vi "Obtain Request Events.vi"(8 "error in (no error)":errorcluster, 10 "Create New?":bool) -> (0 "error out":errorcluster, 2 "FlexiFlowInterface Request Events":T1)   [LabVIEW 2024, in "FlexiFlowInterface.lvlib"]
doc: "This VI Obtains/Creates the Requests events that will be used for other modules to communicate with the module that owns this VI. These Requests events will be accessed only via Public API methods for this module.\n\n<b>NOTE</b>: The contents of this VI are automatically generated and modified by the <b>Tools > Delacor > DQMH</b> utilities. Consider using those utilities instead of making your own modifications to this VI.\n_____\nBased on Delacor QMH Project Template 3.1.0.34."
uses:
  FlexiFlowInterface.lvlib
  Request Events--cluster.ctl
  Stop Argument--cluster.ctl
  Show Panel Argument--cluster.ctl
  Hide Panel Argument--cluster.ctl
  Get Module Execution Status Argument--cluster.ctl
  Show Diagram Argument--cluster.ctl
  Change Panel Argument--cluster.ctl
  <vilib>/MGI/Panel Manager/Panel/Panel/Panel.lvclass
  Start Modbus Polling Helper Loop Argument--cluster.ctl
  Sleep Modbus Polling Helper Loop Argument--cluster.ctl
  Wake Connection Helper Loop Argument--cluster.ctl
  Sleep Connection Helper Loop Argument--cluster.ctl
  Initialise Modbus Connections Argument--cluster.ctl
  Read Fmeasure Argument--cluster.ctl
  FlexiFlowDevice--enum.ctl
  Set Modbus Configuration Argument--cluster.ctl
  Modbus TCP Connection Settings--cluster.ctl
  Wink Devices Argument--cluster.ctl
  Read All FlexiFlow Device States Argument--cluster.ctl
  Wink Device Argument--cluster.ctl
  Set Control Function Argument--cluster.ctl
  Modbus Flexi-Flow API/Control Function Values--enum.ctl
  Set Flow Setpoint Argument--cluster.ctl
  Set Backpressure Setpoint Argument--cluster.ctl
  Set Forward Pressure SP Argument--cluster.ctl
  Set Capacity Unit Argument--cluster.ctl
  Capacity unit--text ring.ctl
  Set Flow Capacity Unit Argument--cluster.ctl
  Modbus Flexi-Flow API/Capacity Units (Standard Volume Flow).ctl
  Set Setpoint Slope Argument--cluster.ctl
  Set Counter Settings Argument--cluster.ctl
  Counter Settings--cluster.ctl
  Modbus Flexi-Flow API/Counter Setpoint Mode--enum.ctl
  Modbus Flexi-Flow API/Counter Modes--enum.ctl
  Reset All Device Counters Argument--cluster.ctl
  Read Device User Tag Argument--cluster.ctl
  Set Device User Tag Argument--cluster.ctl
  Read Counter Unit Argument--cluster.ctl
  Set Control Mode Argument--cluster.ctl
  Modbus Flexi-Flow API/Control Mode--enum.ctl
  Get Device Configuration Argument--cluster.ctl
  Modbus Flexi-Flow API/Bronkhorst Flexi-Flow ModbusTCP API.lvlib
  Anode/Anode.lvlib
panel:
  # "NOTE: The contents of this VI are automatically generated and modified by the Tools > Delacor > DQMH utilities. Consider using those utilities instead of making your own modifications to this VI."
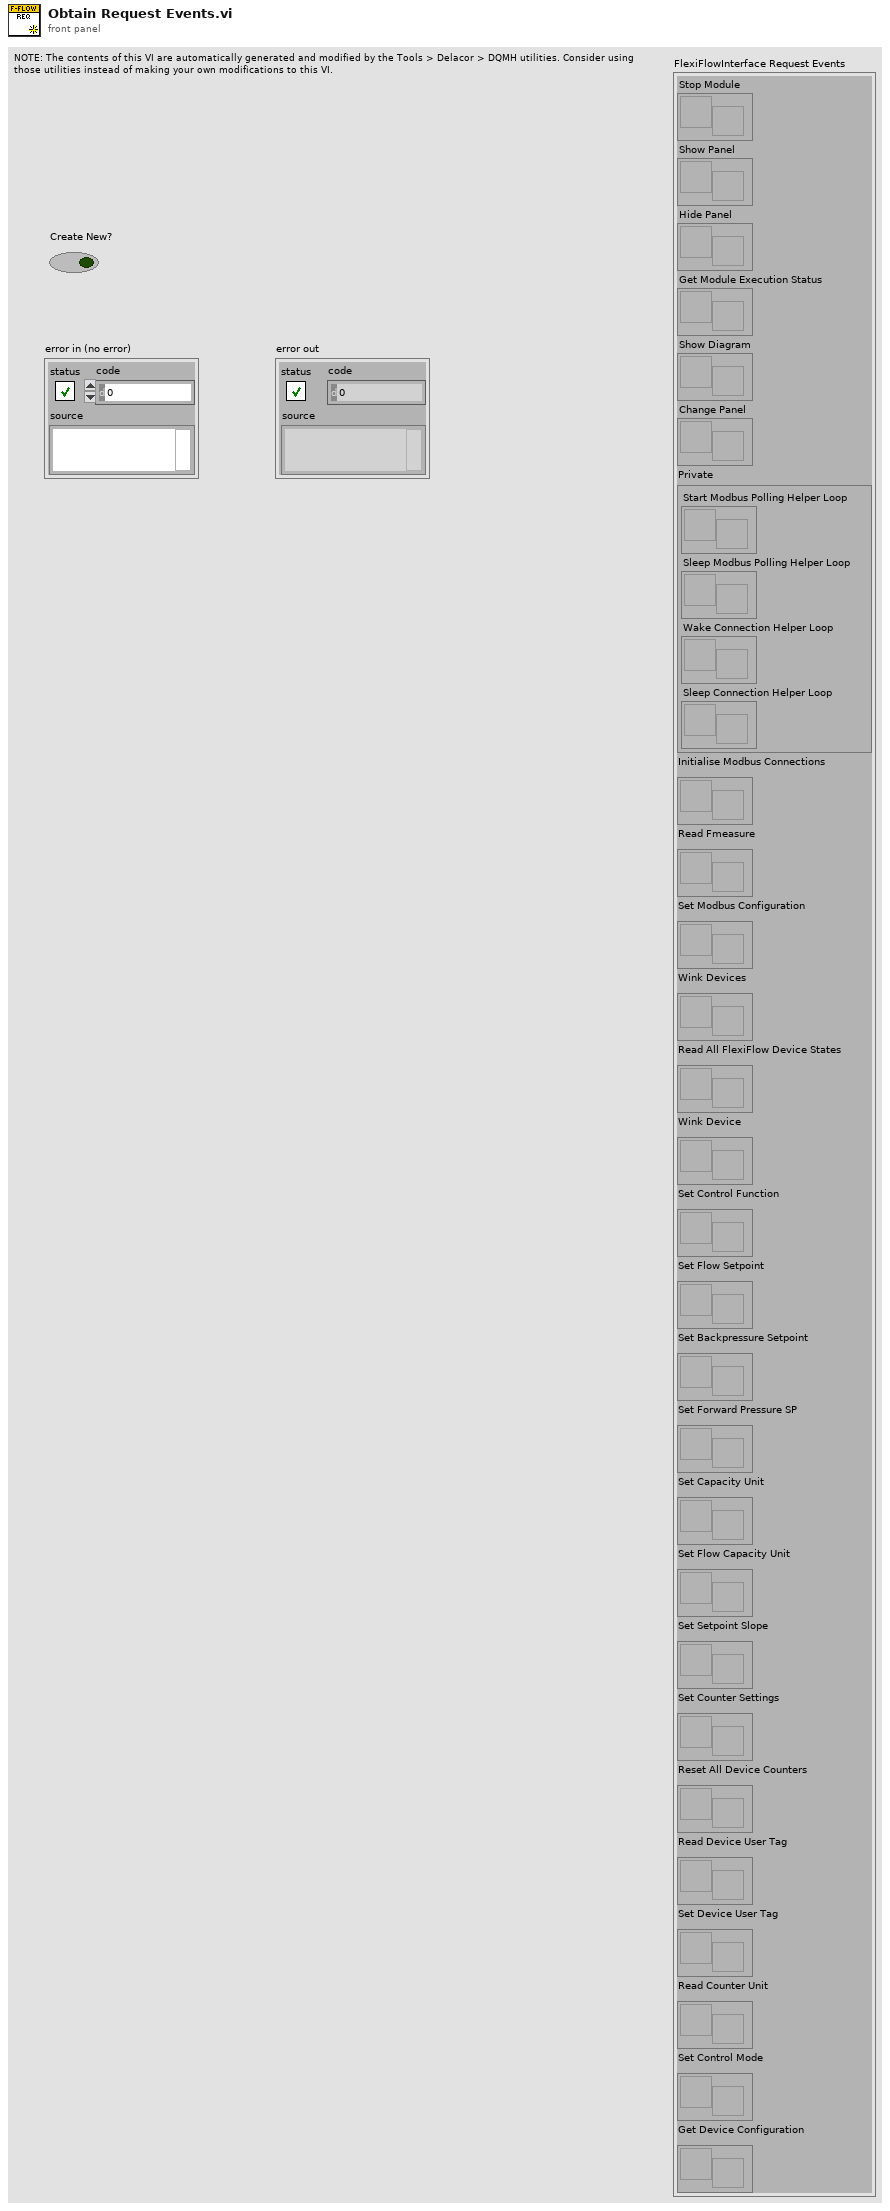
[diagram p1: front panel]
types:
  T1 = typedef "FlexiFlowInterface.lvlib/Request Events--cluster.ctl" = cluster{"Stop Module":refnum<user-event>, "Show Panel":refnum<user-event>, "Hide Panel":refnum<user-event>, "Get Module Execution Status":refnum<user-event>, "Show Diagram":refnum<user-event>, "Change Panel":refnum<user-event>, "Private":cluster{"Start Modbus Polling Helper Loop":refnum<user-event>, "Sleep Modbus Polling Helper Loop":refnum<user-event>, "Wake Connection Helper Loop":refnum<user-event>, "Sleep Connection Helper Loop":refnum<user-event>}, "Initialise Modbus Connections":refnum<user-event>, "Read Fmeasure":refnum<user-event>, "Set Modbus Configuration":refnum<user-event>, "Wink Devices":refnum<user-event>, "Read All FlexiFlow Device States":refnum<user-event>, "Wink Device":refnum<user-event>, "Set Control Function":refnum<user-event>, "Set Flow Setpoint":refnum<user-event>, "Set Backpressure Setpoint":refnum<user-event>, "Set Forward Pressure SP":refnum<user-event>, "Set Capacity Unit":refnum<user-event>, "Set Flow Capacity Unit":refnum<user-event>, "Set Setpoint Slope":refnum<user-event>, "Set Counter Settings":refnum<user-event>, "Reset All Device Counters":refnum<user-event>, "Read Device User Tag":refnum<user-event>, "Set Device User Tag":refnum<user-event>, "Read Counter Unit":refnum<user-event>, "Set Control Mode":refnum<user-event>, "Get Device Configuration":refnum<user-event>}
  T2 = typedef "FlexiFlowInterface.lvlib/Sleep Connection Helper Loop Argument--cluster.ctl" = cluster{"Boolean":bool}
  T3 = typedef "FlexiFlowInterface.lvlib/Wake Connection Helper Loop Argument--cluster.ctl" = cluster{"Boolean":bool}
  T4 = typedef "FlexiFlowInterface.lvlib/Get Device Configuration Argument--cluster.ctl" = cluster{"Device":T5}
  T5 = typedef "FlexiFlowInterface.lvlib/FlexiFlowDevice--enum.ctl" = enum16{"Hydrogen Inlet", "Nitrogen Inlet", "Cathode Outlet", "Anode Outlet"}
  T6 = typedef "FlexiFlowInterface.lvlib/Set Control Mode Argument--cluster.ctl" = cluster{"Device":T5, "Control Mode":T7}
  T7 = typedef "Bronkhorst Flexi-Flow ModbusTCP API.lvlib/Control Mode--enum.ctl" = u16
  T8 = typedef "FlexiFlowInterface.lvlib/Read Counter Unit Argument--cluster.ctl" = cluster{"Device":T5}
  T9 = typedef "FlexiFlowInterface.lvlib/Set Device User Tag Argument--cluster.ctl" = cluster{"Device":T5, "User Tag":string}
  T10 = typedef "FlexiFlowInterface.lvlib/Read Device User Tag Argument--cluster.ctl" = cluster{"Device":T5}
  T11 = typedef "FlexiFlowInterface.lvlib/Reset All Device Counters Argument--cluster.ctl" = cluster{"Boolean":bool}
  T12 = typedef "FlexiFlowInterface.lvlib/Set Counter Settings Argument--cluster.ctl" = cluster{"Device":T5, "Counter Settings":T13}
  T13 = typedef "FlexiFlowInterface.lvlib/Counter Settings--cluster.ctl" = cluster{"Counter Setpoint Mode":T14, "Counter Limit":sgl, "Unit":string, "Counter Mode":T15, "Counter New Setpoint":u16}
  T14 = typedef "Bronkhorst Flexi-Flow ModbusTCP API.lvlib/Counter Setpoint Mode--enum.ctl" = enum16{"No setpoint change (default)", "Change setpoint to Counter new setpoint"}
  T15 = typedef "Bronkhorst Flexi-Flow ModbusTCP API.lvlib/Counter Modes--enum.ctl" = enum16{"Counter off (default)", "Counting up continuously", "Counting up until limit reached"}
  T16 = typedef "FlexiFlowInterface.lvlib/Set Setpoint Slope Argument--cluster.ctl" = cluster{"Setpoint Slope":u16, "Device":T5}
  T17 = typedef "FlexiFlowInterface.lvlib/Set Flow Capacity Unit Argument--cluster.ctl" = cluster{"Device":T5, "Standard Volume Flow":T18}
  T18 = typedef "Bronkhorst Flexi-Flow ModbusTCP API.lvlib/Capacity Units (Standard Volume Flow).ctl" = u16
  T19 = typedef "FlexiFlowInterface.lvlib/Set Capacity Unit Argument--cluster.ctl" = cluster{"Device":T5, "Mass Flow":T20}
  T20 = typedef "Anode.lvlib/Capacity unit--text ring.ctl" = u16
  T21 = typedef "FlexiFlowInterface.lvlib/Set Forward Pressure SP Argument--cluster.ctl" = cluster{"Device":T5, "Pressure SP":dbl}
  T22 = typedef "FlexiFlowInterface.lvlib/Set Backpressure Setpoint Argument--cluster.ctl" = cluster{"Device":T5, "Backpressure SP":dbl}
  T23 = typedef "FlexiFlowInterface.lvlib/Set Flow Setpoint Argument--cluster.ctl" = cluster{"Device":T5, "Setpoint Value":dbl}
  T24 = typedef "FlexiFlowInterface.lvlib/Set Control Function Argument--cluster.ctl" = cluster{"Device":T5, "Function":T25}
  T25 = typedef "Bronkhorst Flexi-Flow ModbusTCP API.lvlib/Control Function Values--enum.ctl" = enum16{"Flow", "Upstream pressure", "Downstream pressure", "Flow with upstream pressure limit", "Flow with downstream pressure limit", "Upstream pressure with flow limit", "Downstream pressure with flow limit"}
  T26 = typedef "FlexiFlowInterface.lvlib/Wink Device Argument--cluster.ctl" = cluster{"Device":T5}
  T27 = typedef "FlexiFlowInterface.lvlib/Read All FlexiFlow Device States Argument--cluster.ctl" = cluster{"Boolean":bool}
  T28 = typedef "FlexiFlowInterface.lvlib/Wink Devices Argument--cluster.ctl" = cluster{"Boolean":bool}
  T29 = typedef "FlexiFlowInterface.lvlib/Set Modbus Configuration Argument--cluster.ctl" = cluster{"Device":T5, "Modbus TCP Connection":T30}
  T30 = typedef "FlexiFlowInterface.lvlib/Modbus TCP Connection Settings--cluster.ctl" = cluster{"Label":string, "Slave ID (255)":u8, "IP Address":string, "Port (502)":u16, "Timeout (10000)":i32}
  T31 = typedef "FlexiFlowInterface.lvlib/Read Fmeasure Argument--cluster.ctl" = cluster{"Device":T5}
  T32 = typedef "FlexiFlowInterface.lvlib/Initialise Modbus Connections Argument--cluster.ctl" = cluster{"Boolean":bool}
  T33 = typedef "FlexiFlowInterface.lvlib/Sleep Modbus Polling Helper Loop Argument--cluster.ctl" = cluster{"Boolean":bool}
  T34 = typedef "FlexiFlowInterface.lvlib/Start Modbus Polling Helper Loop Argument--cluster.ctl" = cluster{"Boolean":bool}
  T35 = typedef "FlexiFlowInterface.lvlib/Change Panel Argument--cluster.ctl" = cluster{"New Panel":refnum<class "Panel.lvclass">}
  T36 = typedef "FlexiFlowInterface.lvlib/Hide Panel Argument--cluster.ctl" = cluster{"Hide Panel?":bool}
  T37 = typedef "FlexiFlowInterface.lvlib/Show Panel Argument--cluster.ctl" = cluster{"Show Panel?":bool}
  T38 = typedef "FlexiFlowInterface.lvlib/Show Diagram Argument--cluster.ctl" = cluster{"Debug?":bool}
  T39 = typedef "FlexiFlowInterface.lvlib/Get Module Execution Status Argument--cluster.ctl" = cluster{"Running?":bool}
  T40 = typedef "FlexiFlowInterface.lvlib/Stop Argument--cluster.ctl" = cluster{"Origin":string, "Exit via Stop Module Req?":bool, "Wait for Module to stop?":bool}
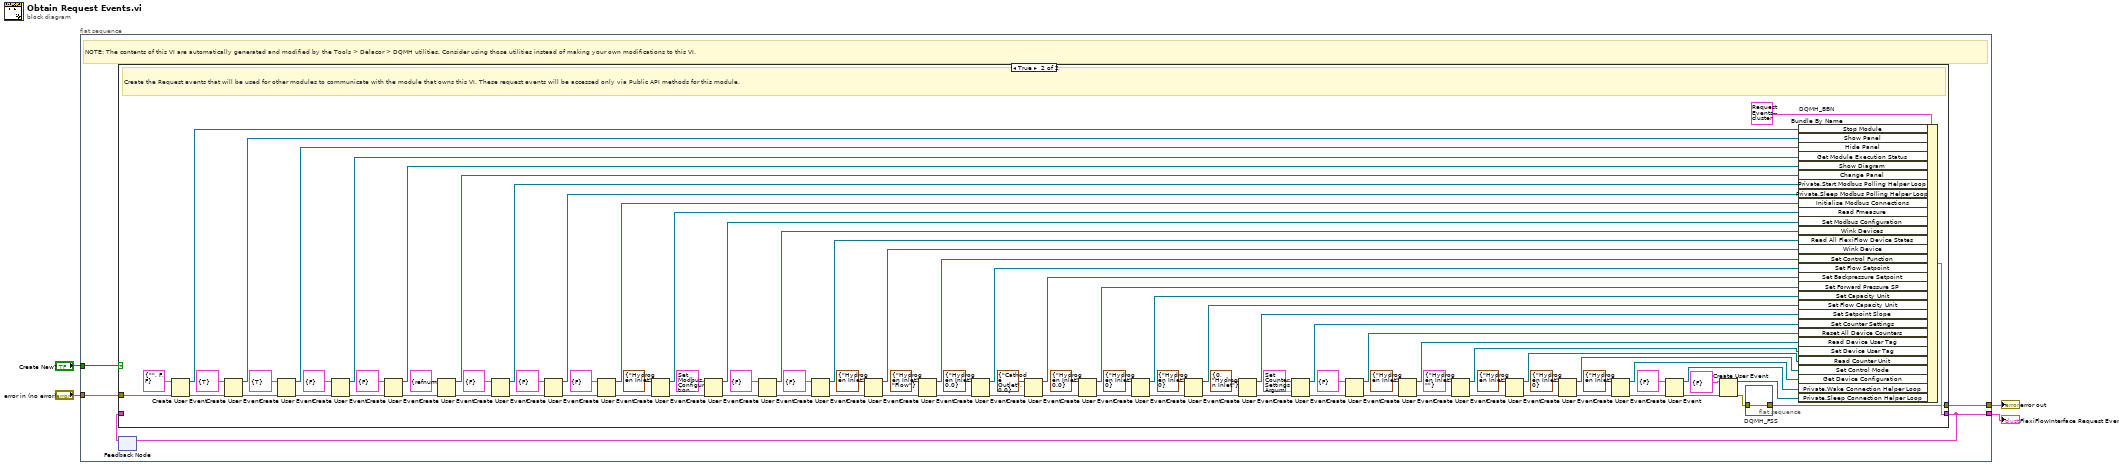
[diagram p0: block diagram]
diagram:
  n1 = flat-sequence {
    tunnel: [w9] -> w4
    tunnel: "error in (no error)" -> [w8]
    tunnel: [w6] -> w2
    tunnel: "Create New?" -> [w5]
    frame #0 {
      # "NOTE: The contents of this VI are automatically generated and modified by the Tools > Delacor > DQMH utilities. Consider using those utilities instead of making your own modifications to this VI."
      n2 = feedback #1() -> (w7:T1)  [unwired: 1 in]
      n3 = case shown="True" w5 {
        tunnel: [w10 w95] -> w9
        tunnel: w8 -> [w10 w105]
        tunnel: [w11 w102] -> w6
        tunnel: w7 -> [w11 _]
        frame False {
          # "Obtain the Request events that were created in a previous call to this VI."
        }
        frame True {
          # "Create the Request events that will be used for other modules to communicate with the module that owns this VI. These request events will be accessed only via Public API methods for this module."
          n4 = Create User Event(user event datatype=T40 {"Origin"="", "Exit via Stop Module Req?"=FALSE, "Wait for Module to stop?"=FALSE} ("Stop Argument"), error in=w105) -> (user event=w103:refnum<user-event>, error out=w100:errorcluster)
          n5 = Create User Event(user event datatype=T37 {"Show Panel?"=TRUE} ("Show Panel Argument"), error in=w100) -> (user event=w99:refnum<user-event>, error out=w98:errorcluster)
          n6 = Create User Event(user event datatype=T36 {"Hide Panel?"=TRUE} ("Hide Panel Argument"), error in=w98) -> (user event=w97:refnum<user-event>, error out=w96:errorcluster)
          n7 = Create User Event(user event datatype=T39 {"Running?"=FALSE} ("Get Module Execution Status Argument"), error in=w96) -> (user event=w93:refnum<user-event>, error out=w94:errorcluster)
          n8 = Create User Event(user event datatype=T38 {"Debug?"=FALSE} ("Show Diagram Argument"), error in=w94) -> (user event=w90:refnum<user-event>, error out=w91:errorcluster)
          n9 = Create User Event(user event datatype=T35 {"New Panel"=refnum} ("Change Panel Argument"), error in=w91) -> (user event=w85:refnum<user-event>, error out=w86:errorcluster)
          n10 = Create User Event(user event datatype=T34 {"Boolean"=FALSE} ("Start Modbus Polling Helper Loop Argument"), error in=w86) -> (user event=w82:refnum<user-event>, error out=w83:errorcluster)
          n11 = Create User Event(user event datatype=T33 {"Boolean"=FALSE} ("Sleep Modbus Polling Helper Loop Argument"), error in=w83) -> (user event=w79:refnum<user-event>, error out=w80:errorcluster)
          n12 = Create User Event(user event datatype=T32 {"Boolean"=FALSE} ("Initialise Modbus Connections Argument"), error in=w80) -> (user event=w76:refnum<user-event>, error out=w77:errorcluster)
          n13 = Create User Event(user event datatype=T31 {"Device"=enum."Hydrogen Inlet"} ("Read Device State Argument"), error in=w77) -> (user event=w73:refnum<user-event>, error out=w74:errorcluster)
          n14 = Create User Event(user event datatype=T29 {"Device"=enum."Hydrogen Inlet", "Modbus TCP Connection"={"Label"="", "Slave ID (255)"=255, "IP Address"="", "Port (502)"=502, "Timeout (10000)"=10000}} ("Set Modbus Configuration Argument"), error in=w74) -> (user event=w70:refnum<user-event>, error out=w71:errorcluster)
          n15 = Create User Event(user event datatype=T28 {"Boolean"=FALSE} ("Wink Devices Argument"), error in=w71) -> (user event=w67:refnum<user-event>, error out=w68:errorcluster)
          n16 = Create User Event(user event datatype=T27 {"Boolean"=FALSE} ("Read All FlexiFlow Device States Argument"), error in=w68) -> (user event=w64:refnum<user-event>, error out=w65:errorcluster)
          n17 = Create User Event(user event datatype=T26 {"Device"=enum."Hydrogen Inlet"} ("Wink Device Argument"), error in=w65) -> (user event=w61:refnum<user-event>, error out=w62:errorcluster)
          n18 = Create User Event(user event datatype=T24 {"Device"=enum."Hydrogen Inlet", "Function"=enum."Flow"} ("Set Control Function Argument"), error in=w62) -> (user event=w58:refnum<user-event>, error out=w59:errorcluster)
          n19 = Create User Event(user event datatype=T23 {"Device"=enum."Hydrogen Inlet", "Setpoint Value"=0.0} ("Set Control Value SP Argument"), error in=w59) -> (user event=w55:refnum<user-event>, error out=w56:errorcluster)
          n20 = Create User Event(user event datatype=T22 {"Device"=enum."Cathode Outlet", "Backpressure SP"=0.0} ("Set Backpressure Setpoint Argument"), error in=w56) -> (user event=w52:refnum<user-event>, error out=w53:errorcluster)
          n21 = Create User Event(user event datatype=T21 {"Device"=enum."Hydrogen Inlet", "Pressure SP"=0.0} ("Set Forward Pressure SP Argument"), error in=w53) -> (user event=w49:refnum<user-event>, error out=w50:errorcluster)
          n22 = Create User Event(user event datatype=T19 {"Device"=enum."Hydrogen Inlet", "Mass Flow"=0} ("Set Capacity Unit Argument"), error in=w50) -> (user event=w46:refnum<user-event>, error out=w47:errorcluster)
          n23 = Create User Event(user event datatype=T17 {"Device"=enum."Hydrogen Inlet", "Standard Volume Flow"=0} ("Set Flow Capacity Unit Argument"), error in=w47) -> (user event=w43:refnum<user-event>, error out=w44:errorcluster)
          n24 = Create User Event(user event datatype=T16 {"Setpoint Slope"=0, "Device"=enum."Hydrogen Inlet"} ("Set Setpoint Slope Argument"), error in=w44) -> (user event=w40:refnum<user-event>, error out=w41:errorcluster)
          n25 = Create User Event(user event datatype=T12 {"Device"=enum."Hydrogen Inlet", "Counter Settings"={"Counter Setpoint Mode"=enum."No setpoint change (default)", "Counter Limit"=0.0, "Unit"="ls", "Counter Mode"=enum."Counter off (default)", "Counter New Setpoint"=0}} ("Set Counter Settings Argument"), error in=w41) -> (user event=w37:refnum<user-event>, error out=w38:errorcluster)
          n26 = Create User Event(user event datatype=T11 {"Boolean"=FALSE} ("Reset All Device Counters Argument"), error in=w38) -> (user event=w34:refnum<user-event>, error out=w35:errorcluster)
          n27 = Create User Event(user event datatype=T10 {"Device"=enum."Hydrogen Inlet"} ("Read Device User Tag Argument"), error in=w35) -> (user event=w31:refnum<user-event>, error out=w32:errorcluster)
          n28 = Create User Event(user event datatype=T9 {"Device"=enum."Hydrogen Inlet", "User Tag"=""} ("Set Device User Tag Argument"), error in=w32) -> (user event=w28:refnum<user-event>, error out=w29:errorcluster)
          n29 = Create User Event(user event datatype=T8 {"Device"=enum."Hydrogen Inlet"} ("Read Counter Unit Argument"), error in=w29) -> (user event=w25:refnum<user-event>, error out=w26:errorcluster)
          n30 = Create User Event(user event datatype=T6 {"Device"=enum."Hydrogen Inlet", "Control Mode"=0} ("Set Control Mode Argument"), error in=w26) -> (user event=w22:refnum<user-event>, error out=w23:errorcluster)
          n31 = Create User Event(user event datatype=T4 {"Device"=enum."Hydrogen Inlet"} ("Get Device Configuration Argument"), error in=w23) -> (user event=w19:refnum<user-event>, error out=w20:errorcluster)
          n32 = Create User Event(user event datatype=T3 {"Boolean"=FALSE} ("Wake Connection Helper Loop Argument"), error in=w20) -> (user event=w16:refnum<user-event>, error out=w17:errorcluster)
          n33 = Create User Event(user event datatype=T2 {"Boolean"=FALSE} ("Sleep Connection Helper Loop Argument"), error in=w17) -> (user event=w13:refnum<user-event>, error out=w14:errorcluster)
          n34 = flat-sequence "DQMH_FSS" {
            tunnel: w14 -> [w106]
            tunnel: [w106] -> w95
            frame #0 {
            }
          }
          n35 = Bundle By Name "DQMH_BBN"(cluster=T1 {"Stop Module"=refnum, "Show Panel"=refnum, "Hide Panel"=refnum, "Get Module Execution Status"=refnum, "Show Diagram"=refnum, "Change Panel"=refnum, "Private"={"Start Modbus Polling Helper Loop"=refnum, "Sleep Modbus Polling Helper Loop"=refnum, "Wake Connection Helper Loop"=refnum, "Sleep Connection Helper Loop"=refnum}, "Initialise Modbus Connections"=refnum, "Read Fmeasure"=refnum, "Set Modbus Configuration"=refnum, "Wink Devices"=refnum, "Read All FlexiFlow Device States"=refnum, "Wink Device"=refnum, "Set Control Function"=refnum, "Set Flow Setpoint"=refnum, "Set Backpressure Setpoint"=refnum, "Set Forward Pressure SP"=refnum, "Set Capacity Unit"=refnum, "Set Flow Capacity Unit"=refnum, "Set Setpoint Slope"=refnum, "Set Counter Settings"=refnum, "Reset All Device Counters"=refnum, "Read Device User Tag"=refnum, "Set Device User Tag"=refnum, "Read Counter Unit"=refnum, "Set Control Mode"=refnum, "Get Device Configuration"=refnum} ("output cluster"), "Stop Module"=w103, "Show Panel"=w99, "Hide Panel"=w97, "Get Module Execution Status"=w93, "Show Diagram"=w90, "Change Panel"=w85, "Private.Start Modbus Polling Helper Loop"=w82, "Private.Sleep Modbus Polling Helper Loop"=w79, "Initialise Modbus Connections"=w76, "Read Fmeasure"=w73, "Set Modbus Configuration"=w70, "Wink Devices"=w67, "Read All FlexiFlow Device States"=w64, "Wink Device"=w61, "Set Control Function"=w58, "Set Flow Setpoint"=w55, "Set Backpressure Setpoint"=w52, "Set Forward Pressure SP"=w49, "Set Capacity Unit"=w46, "Set Flow Capacity Unit"=w43, "Set Setpoint Slope"=w40, "Set Counter Settings"=w37, "Reset All Device Counters"=w34, "Read Device User Tag"=w31, "Set Device User Tag"=w28, "Read Counter Unit"=w25, "Set Control Mode"=w22, "Get Device Configuration"=w19, "Private.Wake Connection Helper Loop"=w16, "Private.Sleep Connection Helper Loop"=w13) -> (w102:T1)
        }
      }
      n36 = feedback-in #1(w6) -> ()
    }
  }
  "FlexiFlowInterface Request Events" <- w2
  "error out" <- w4
